vi "Get Table.vi"(7 "Sheet Name in":string, 8 "error in":errorcluster, 10 "Table Name":string, 11 "SpreadsheetDoc in":refnum<k24>) -> (0 "error out":errorcluster, 2 "Table":refnum<k24>, 3 "SpreadsheetDoc out":refnum<k24>, 5 "Sheet Name out":string)   [LabVIEW 2019, in "Open Xml.lvlib"]
uses:
  Open Xml.lvlib
  D:/git/Open-Xml-LabVIEW/Source/DocumentFormat.OpenXml.dll
  DocumentFormat.OpenXml.dll
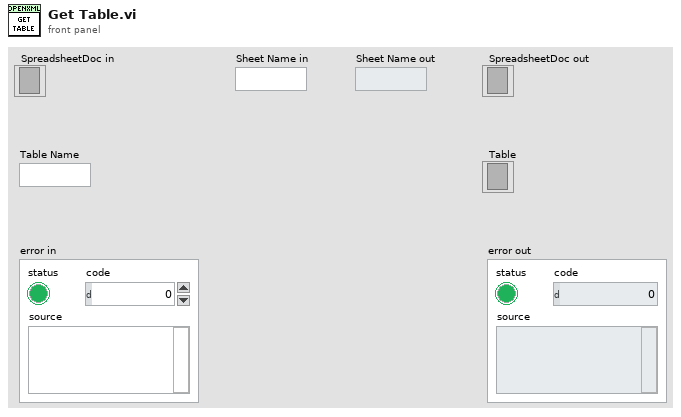
[diagram p1: front panel]
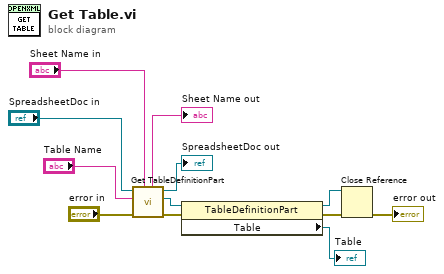
[diagram p0: block diagram]
diagram:
  n1 = call "Get TableDefinitionPart.vi"("Sheet Name"="Sheet Name in", "error in"="error in", "Table Name"="Table Name", "SpreadsheetDoc in"="SpreadsheetDoc in") -> ("error out"=w6:errorcluster, "TableDefinitionPart"=w7:refnum<k24>, "SpreadsheetDo out"=→"SpreadsheetDoc out":refnum<k24>, "Sheet Name"=→"Sheet Name out":string)  [unwired: 4 in]
  n2 = property class="TableDefinitionPart"(reference=w7, error in=w6) -> (reference out=w5:refnum<k24>, error out=w3:errorcluster, "Table"=→"Table":refnum<k24>)
  n3 = Close Reference(reference=w5, error in (no error)=w3) -> (error out=→"error out":errorcluster)
